vi "Exposure-Analyze.vi"(0 "Exposure parameters":T2, 1 "SPL Log In":cluster{"t0":dbl, "dt (min)":dbl, "SPL":dbl[][]}, 5 "Runtime Data":T1, 9 "AI Waveforms":dbl[][](array[numeric]), 11 "error in (no error)":errorcluster, 12 "Sampling Rate (Hz)":dbl) -> (3 "SPL Log Out":cluster{dbl, "Buffer length (s)":dbl, dbl[][]}, 4 "Waveform":waveform(dbl)[](array[waveform]), 6 "Spectrum":waveform(dbl)[](array[waveform]), 8 "PT SPL":dbl[](array[numeric]), 15 "error out":errorcluster)   [LabVIEW 2020]
uses:
  Typedefs/Exposure Parameters.ctl
  Typedefs/Exposure-Runtime Data.ctl
  epl-vi-lib/Utility VIs/Math VIs/dB to Linear (scalar).vi
  epl-vi-lib/Utility VIs/Math VIs/FFT x(t) to dB,Degrees (1D).vi
  epl-vi-lib/Utility VIs/Math VIs/dB to Linear (1D).vi
  epl-vi-lib/Utility VIs/Math VIs/Linear to dB (scalar).vi
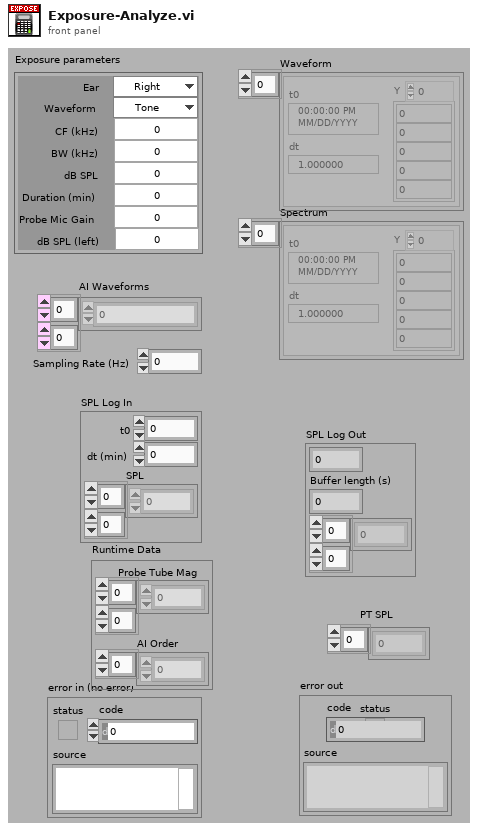
[diagram p1: front panel]
types:
  T1 = typedef "Exposure-Runtime Data.ctl" = cluster{"Probe Tube Mag":dbl[][], "AI Order":i32[]}
  T2 = typedef "Exposure Parameters.ctl" = cluster{"Probe Mic Gain":dbl, "Waveform":enum16{"Tone", "Noise"}, "CF (kHz)":dbl, "BW (kHz)":dbl, "Ear":enum16{"Right", "Left", "Binaural"}, "Duration (min)":dbl, "dB SPL":dbl, "dB SPL (left)":dbl}
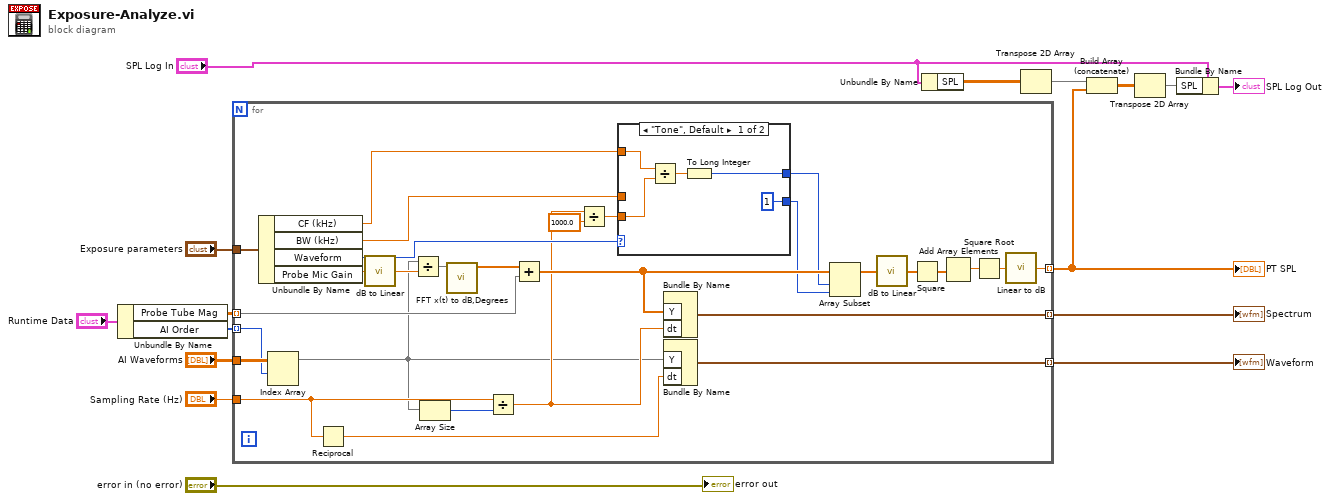
[diagram p0: block diagram]
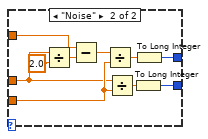
[diagram p2: hidden frame]
diagram:
  n1 = Unbundle By Name("Runtime Data") -> ("Probe Tube Mag"=w9:dbl[][], "AI Order"=w8:i32[])
  n2 = for {
    tunnel: "Exposure parameters" -> [w43]
    tunnel: "Sampling Rate (Hz)" -> [w40]
    tunnel: "AI Waveforms" -> [w21]
    tunnel: [w20] -> w6 mode=indexing
    tunnel: [w23] -> w12 mode=indexing
    tunnel: [w22] -> w11 mode=indexing
    tunnel: w9 -> [w19] mode=indexing
    tunnel: w8 -> [w17] mode=indexing
    n3 = Unbundle By Name(w43) -> ("CF (kHz)"=w29:dbl, "BW (kHz)"=w30:dbl, "Waveform"=w32:enum16{"Tone", "Noise"}, "Probe Mic Gain"=w42:dbl)
    n4 = Index Array(array=w21, index (row)=w17) -> (element=w18:dbl[])  [unwired: 1 in]
    n5 = Reciprocal(x=w40) -> (1/x=w41:dbl)
    n6 = call-poly "dB to Linear.vi"("dB"=w42) -> ("linear"=w45:dbl)
    n7 = Divide(x=w18, y=w45) -> (x/y=w44:dbl[])
    n8 = Array Size(array=w18) -> (size(s)=w39:i32)
    n9 = call-poly "FFT x(t) to dB,Degrees.vi"("X"=w44) -> ("+Freq. Mag of FFT (dB rms)"=w34:dbl[])  [unwired: 8 in, 2 out]
    n10 = Divide(x=w40, y=w39) -> (x/y=w31:dbl)
    n11 = Add(x=w34, y=w19) -> (x+y=w33:dbl[])
    n12 = Divide(x=w31, y=1000.0) -> (x/y=w25:dbl)
    n13 = case shown="\"Tone\", Default" w32 {
      tunnel: w25 -> [w49 w56]
      tunnel: w30 -> [_ w51]
      tunnel: w29 -> [w50 w59]
      tunnel: [w47 w53] -> w28
      tunnel: [1 w52] -> w27
      frame "Tone", Default {
        n14 = Divide(x=w50, y=w49) -> (x/y=w48:dbl)
        n15 = To Long Integer(number=w48) -> (32bit integer=w47:i32)
      }
      frame "Noise" {
        n16 = Divide(x=w51, y=2.0) -> (x/y=w58:dbl)
        n17 = Subtract(x=w59, y=w58) -> (x-y=w57:dbl)
        n18 = Divide(x=w57, y=w56) -> (x/y=w55:dbl)
        n19 = Divide(x=w51, y=w56) -> (x/y=w54:dbl)
        n20 = To Long Integer(number=w54) -> (32bit integer=w52:i32)
        n21 = To Long Integer(number=w55) -> (32bit integer=w53:i32)
      }
    }
    n22 = Bundle By Name("Y"=w33, "dt"=w31) -> (w23:waveform(dbl))  [unwired: 1 in]
    n23 = Bundle By Name("Y"=w18, "dt"=w41) -> (w22:waveform(dbl))  [unwired: 1 in]
    n24 = Array Subset(array=w33, index=w28, length=w27) -> (w26:dbl[])
    n25 = call-poly "dB to Linear.vi"("dB"=w26) -> ("linear"=w38:dbl[])
    n26 = Square(x=w38) -> (x^2=w37:dbl[])
    n27 = Add Array Elements(numeric array=w37) -> (sum=w36:dbl)
    n28 = Square Root(x=w36) -> (sqrt(x)=w35:dbl)
    n29 = call-poly "Linear to dB.vi"("Linear"=w35) -> ("dB"=w20:dbl)
  }
  "PT SPL" <- w6
  "Spectrum" <- w12
  "Waveform" <- w11
  n30 = Unbundle By Name("SPL Log In") -> ("SPL"=w7:dbl[][])
  n31 = Transpose 2D Array(2D array=w7) -> (transposed array=w2:dbl[][])
  n32 = Build Array (concatenate)(w2, w6) -> (w5:dbl[][])
  n33 = Transpose 2D Array(2D array=w5) -> (transposed array=w1:dbl[][])
  n34 = Bundle By Name(cluster="SPL Log In", "SPL"=w1) -> (→"SPL Log Out":cluster{"t0":dbl, "dt (min)":dbl, "SPL":dbl[][]})
  "error out" <- "error in (no error)"
